vi "Disconnect All.vi"(8 "error in (no error)":errorcluster, 11 "NI-SWITCH Consumer in":refnum<class "NI-SWITCH Consumer.lvclass">) -> (0 "error out":errorcluster, 3 "NI-SWITCH Consumer out":refnum<class "NI-SWITCH Consumer.lvclass">)   [LabVIEW 2020, in "NI-SWITCH Messaging.lvlib" / "NI-SWITCH Consumer.lvclass"]
uses:
  NI-SWITCH Consumer.lvclass
  NI-SWITCH Consumer.lvclass/NI-SWITCH Consumer.ctl
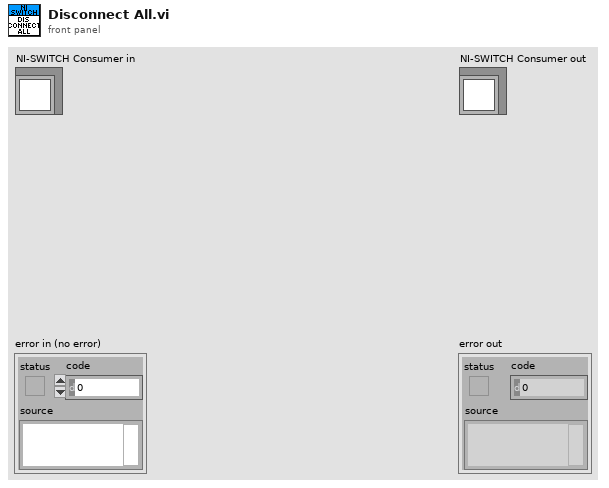
[diagram p1: front panel]
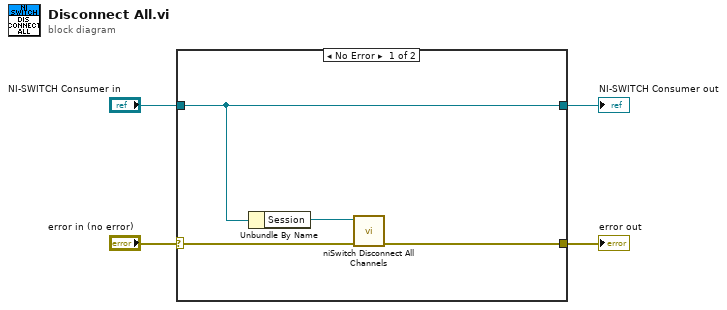
[diagram p0: block diagram]
diagram:
  n1 = case shown="No Error" "error in (no error)" {
    selector: "error in (no error)" -> [w6 w10]
    tunnel: [w5 w10] -> w3
    tunnel: [w8 w9] -> w1
    tunnel: "NI-SWITCH Consumer in" -> [w8 w9]
    frame No Error {
      n2 = Unbundle By Name(w8) -> ("Session"=w7:refnum<k15>)
      n3 = call <instrlib>:"niSwitch Disconnect All Channels.vi"("error in (no error)"=w6, "instrument handle"=w7) -> ("error out"=w5:errorcluster)  [unwired: 8 in, 1 out]
    }
    frame Error {
    }
  }
  "error out" <- w3
  "NI-SWITCH Consumer out" <- w1
